vi "3st body(json).vi"(0 "third test item name":string, 1 "file path (dialog if empty)":path caption="文件路径 （空时为对话框）", 2 "ABS?":bool, 3 "Points":dbl[](array[numeric]), 5 "second result":string, 7 "single spec":dbl[](array[numeric]), 9 "TDD spec":string, 11 "SN":string, 12 "limit type":enum16{"上限", "下限"}(ring), 13 "TDD?":bool, 14 "StatusRef":refnum<vi>) -> (6 "OutPutXml":string)   [LabVIEW 2011]
panel:
  out "all rows":string[][](array[string])
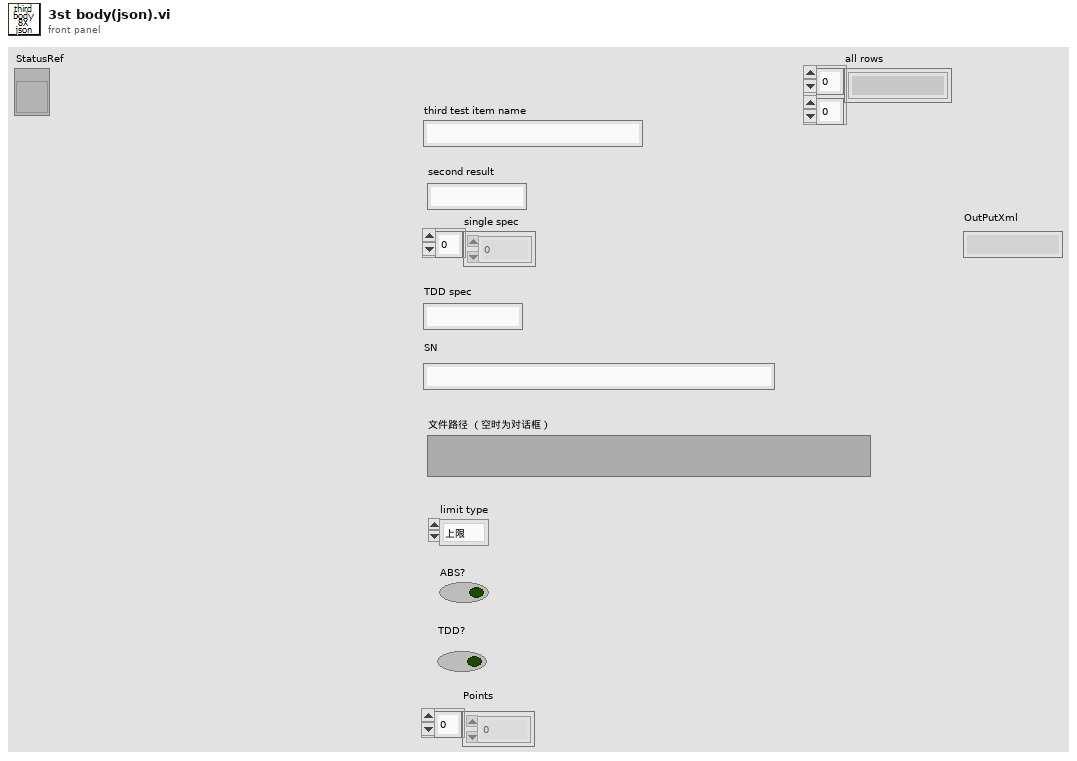
[diagram p1: front panel]
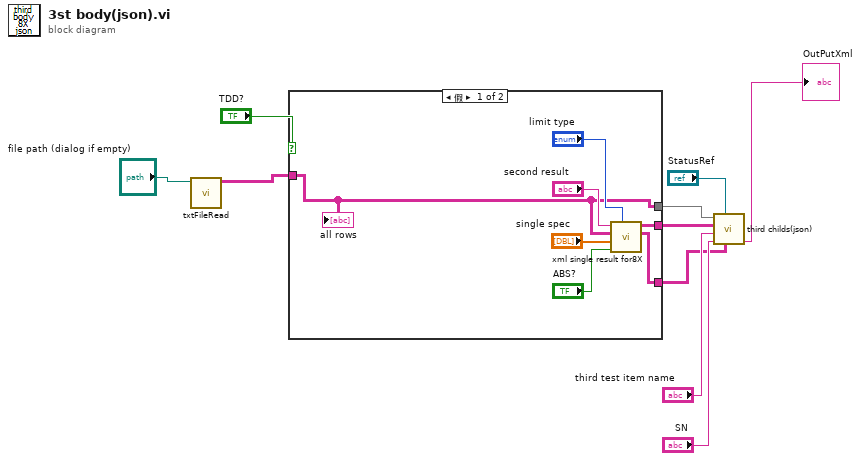
[diagram p0: block diagram]
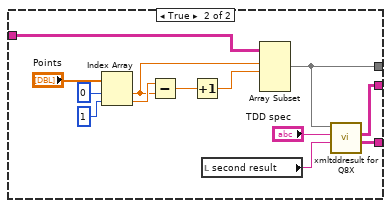
[diagram p2: hidden frame]
diagram:
  n1 = call "txtFileRead.vi"("file path (dialog if empty)"="file path (dialog if empty)") -> ("all rows"=w3:string[][])  [unwired: 10 in]
  n2 = case shown="假" "TDD?" {
    tunnel: w3 -> [w15 w30]
    tunnel: [w15 w22] -> w6
    tunnel: [w12 w19] -> w9
    tunnel: [w11 w18] -> w2
    frame False {
      n3 = call "xml single result for8X.vi"("limitType"="limit type", "abs?"="ABS?", "single spec"="single spec", "dataSource"=w15, "second result"="second result") -> ("pointValue"=w11:string[][], "third result"=w12:string[][])  [unwired: 5 in]
      "all rows" <- w15
    }
    frame True {
      n4 = Index Array(array="Points", index #1=0 ("索引"), index #2=1 ("索引")) -> (element #1=w25:dbl, element #2=w26:dbl)
      n5 = Subtract(x=w26, y=w25) -> (x-y=w24:dbl)
      n6 = Increment(x=w24) -> (x+1=w23:dbl)
      n7 = local read "second result"() -> (w20:string)
      n8 = Array Subset(array=w30, index (row)=w25, length (row)=w23) -> (w22:string[][])  [unwired: 2 in]
      n9 = call "xmltddresult for Q8X.vi"("second result"=w20, "TDD spec"="TDD spec", "TDD array"=w22) -> ("pointValue"=w18:string[][], "TDD third result"=w19:string[][])  [unwired: 7 in]
    }
  }
  n10 = call "third childs(json).vi"("pointSpec"=w2, "StatusRef"="StatusRef", "SN"="SN", "third test item name"="third test item name", "third result"=w9, "all rows"=w6) -> ("thirdChilds"=→"OutPutXml":string)  [unwired: 5 in]
